vi "WOT.vi"(1 "Bring up WOT":bool, 2 "Put down WOT":bool, 3 "Take in ball":bool, 4 "Push out ball":bool) -> (0 "Wheels on Top Speed":dbl)   [LabVIEW 2013]
uses:
  <vilib>/Rock Robotics/WPI/Solenoid/WPI_SolenoidValue.ctl
  <vilib>/Rock Robotics/WPI/Solenoid/WPI_SolenoidSetEnum.vi
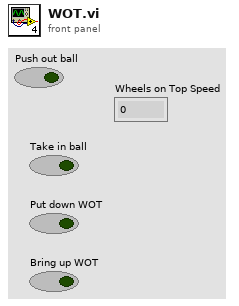
[diagram p1: front panel]
types:
  T1 = typedef "WPI_SolenoidValue.ctl" = enum16{"Off", "On", "Forward", "Reverse"}
  T2 = typedef "WPI_SolenoidDevRef.ctl" = cluster{"DevStatus":errorcluster, "Solenoid Module":T3, "Forward Solenoid Channel":T4, "Reverse Solenoid Channel":T4}
  T3 = typedef "FPGA_TypedefSolenoidModule.ctl" = enum16{"Solenoid Module 1", "Solenoid Module 2"}
  T4 = typedef "WPI_SolenoidChannel.ctl" = enum8{"Solenoid 1", "Solenoid 2", "Solenoid 3", "Solenoid 4", "Solenoid 5", "Solenoid 6", "Solenoid 7", "Solenoid 8", "Invalid"}
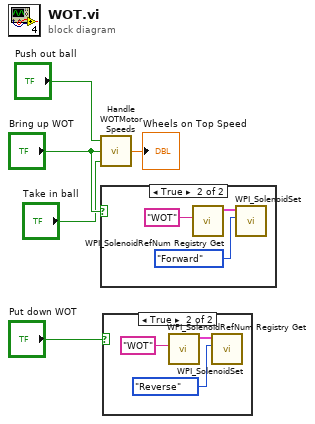
[diagram p0: block diagram]
diagram:
  n1 = call "Handle WOTMotor Speeds.vi"("Take in ball"="Take in ball", "Bring in WOT"="Bring up WOT", "Push out ball"="Push out ball") -> ("Wheels on Top"=→"Wheels on Top Speed":dbl)
  n2 = case shown="True" "Bring up WOT" {
    frame False {
    }
    frame True {
      n3 = call <vilib>:"WPI_SolenoidRefNum Registry Get.vi"("refnum name"="WOT") -> ("SolenoidDevRef"=w7:T2)  [unwired: 9 in, 1 out]
      n4 = call-poly <vilib>:"WPI_SolenoidSet.vi"("Value"=WPI_SolenoidValue."Forward" ("t"), "SolenoidDevRef"=w7) -> ()  [unwired: 8 in, 2 out]
    }
  }
  n5 = case shown="True" "Put down WOT" {
    frame False {
    }
    frame True {
      n6 = call <vilib>:"WPI_SolenoidRefNum Registry Get.vi"("refnum name"="WOT") -> ("SolenoidDevRef"=w10:T2)  [unwired: 9 in, 1 out]
      n7 = call-poly <vilib>:"WPI_SolenoidSet.vi"("Value"=WPI_SolenoidValue."Reverse" ("t"), "SolenoidDevRef"=w10) -> ()  [unwired: 8 in, 2 out]
    }
  }
